vi "findnextw.vi"(0 "Vref":dbl, 1 "next_y":dbl, 3 "index":dbl, 5 "next_x":dbl, 9 "cur_angle":dbl, 12 "cur_x":dbl, 13 "cur_y":dbl) -> (4 "w_left":dbl, 6 "w_right":dbl, 15 "theta":cdb)   [LabVIEW 2015]
uses:
  <vilib>/imath/engines/lvmath2/RunTimeEngine/NodeEndStatement/NIMS_NodeEndStatement_Output.vi
  <instcachedir>/0/NIMS_NodeEndStatement_Output_53EC0D466D134D7ABD903AC30B43404B.lvgen/NIMS_NodeEndStatement_Output_53EC0D466D134D7ABD903AC30B43404B_009.vi
  <instcachedir>/0/NIMS_NodeEndStatement_Output_53EC0D466D134D7ABD903AC30B43404B.lvgen/NIMS_NodeEndStatement_Output_53EC0D466D134D7ABD903AC30B43404B_001.vi
  <vilib>/imath/engines/lvmath2/RunTimeEngine/ErrorHandling/NIMS_Finalize Error.vi
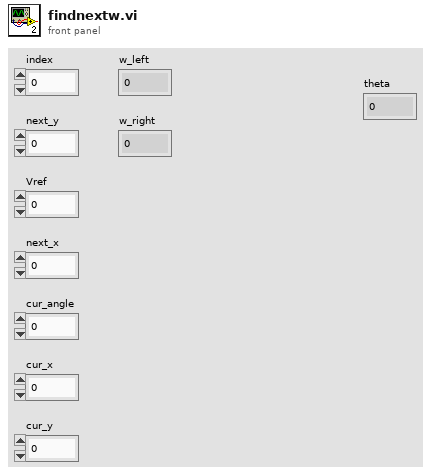
[diagram p1: front panel]
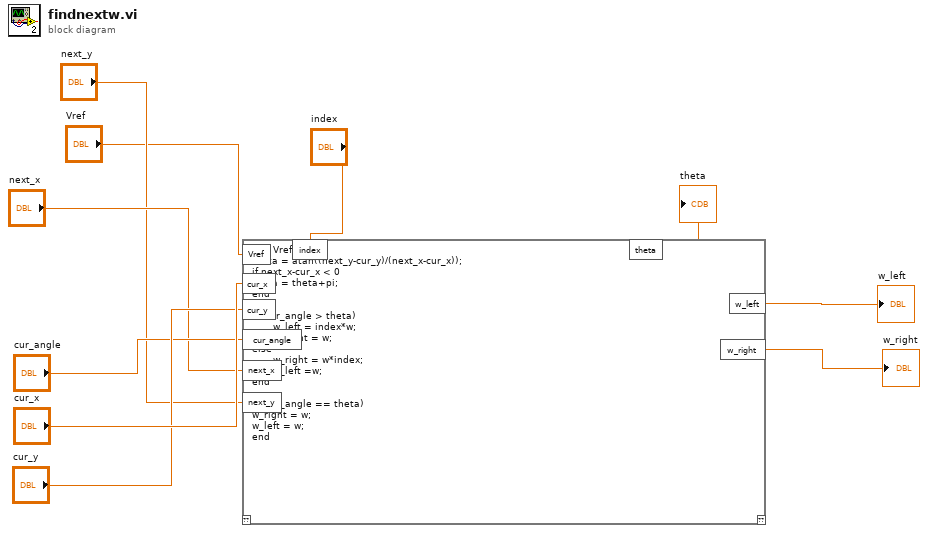
[diagram p0: block diagram]
diagram:
  n1 = mathscript code="w = Vref/0.05;\ntheta = atan((next_y-cur_y)/(next_x-cur_x));\nif next_x-cur_x < 0\ntheta = theta+pi;\nend\n\nif (cur_angle > theta)\n       w_left = index*w;\n       w_right = w;\nelse\n       w_right = w*index;\n       w_left =w;\nend\n\nif (cur_angle == theta)\nw_right = w;\nw_left = w;\nend"("cur_x"="cur_x", "cur_y"="cur_y", "cur_angle"="cur_angle", "next_x"="next_x", "next_y"="next_y", "Vref"="Vref", "index"="index") -> ("w_left"=→"w_left":dbl, "w_right"=→"w_right":dbl, "theta"=→"theta":cdb)  [unwired: 1 in, 1 out]
